vi "example1.vi"() -> ()   [LabVIEW 2010]
panel:
  out "error out":errorcluster
  in  "error in (no error)":errorcluster
  out "remote access":bool
  out "WindowName":string[](array[string])
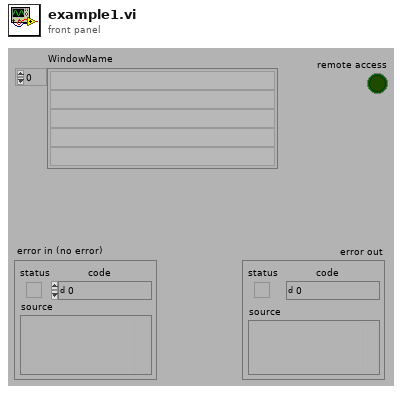
[diagram p1: front panel]
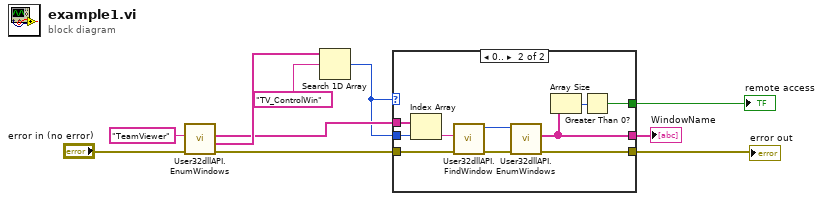
[diagram p0: block diagram]
diagram:
  n1 = call "User32dllAPI.EnumWindows.vi"("error in (no error)"="error in (no error)", "Pattern"="TeamViewer") -> ("error out"=w10:errorcluster, "ClassName"=w8:string[], "WindowName"=w7:string[])  [unwired: 6 in, 1 out]
  n2 = Search 1D Array(1D array=w8, element="TV_ControlWin") -> (index of element=w4:i32)  [unwired: 1 in]
  n3 = case shown="0.." w4 {
    tunnel: w10 -> [w11 w21]
    tunnel: w7 -> [_ w20]
    tunnel: w4 -> [_ w19]
    tunnel: [_ w12] -> w5
    tunnel: [w11 w15] -> w2
    tunnel: [_ w13] -> w3
    frame Default {
    }
    frame 0.. {
      n4 = Index Array(array=w20, index=w19) -> (element=w18:string)
      n5 = call "User32dllAPI.FindWindow.vi"("error in (no error)"=w21, "WindowName"=w18) -> ("error out"=w17:errorcluster, "hWnd"=w16:i32)  [unwired: 8 in]
      n6 = call "User32dllAPI.EnumWindows.vi"("error in (no error)"=w17, "hWnd in (NULL)"=w16) -> ("error out"=w15:errorcluster, "WindowName"=w12:string[])  [unwired: 6 in, 2 out]
      n7 = Array Size(array=w12) -> (size(s)=w14:i32)
      n8 = Greater Than 0?(x=w14) -> (x > 0?=w13:bool)
    }
  }
  "WindowName" <- w5
  "remote access" <- w3
  "error out" <- w2
